vi "Wind Turbine Simulation - Three Cluster.vi"() -> (0 "Cluster":T3)   [LabVIEW 2011]
doc: "This is a cluster for a Wind Turbine template.\n\nAAL 9/09"
uses:
  Controls/File Type.ctl
  Wind Report/Wind Report.lvclass
  SEQ Solution/Controls/Wind Turbine DataRef.ctl
  SEQ Solution/Controls/Wind Turbine Data.ctl
  SEQ Solution/SEQ - Solution.lvlib
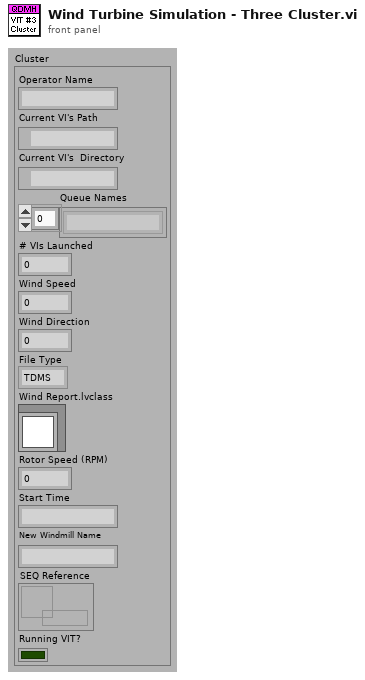
[diagram p1: front panel]
types:
  T1 = typedef "File Type.ctl" = enum16{"TDMS", "TXT"}
  T2 = typedef "SEQ - Solution.lvlib/Wind Turbine DataRef.ctl" = refnum<queue>
  T3 = cluster{"Operator Name":string, "Current VI's Path":path, "Current VI's  Directory":path, "Queue Names":string[], "# VIs Launched":i32, "Wind Speed":dbl, "Wind Direction":dbl, "File Type":T1, "Wind Report.lvclass":refnum<class "Wind Report.lvclass">, "Rotor Speed (RPM)":dbl, "Start Time":string, "New Windmill Name":string, "SEQ Reference":T2, "Running VIT?":bool}
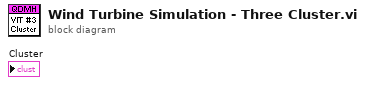
[diagram p0: block diagram]
diagram:
